vi "CheckforDFDToolkit.vi"(8 "error in (no error)":errorcluster) -> (0 "error out":errorcluster, 3 "NI LabVIEW Digital Filter Design Toolkit version":string)   [LabVIEW 2013]
uses:
  <vilib>/nisyscfg/Get Installed Components.vi
  <vilib>/nisyscfg/nisyscfg.lvlib
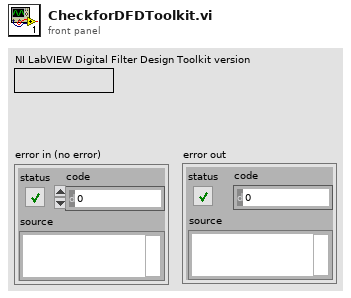
[diagram p1: front panel]
types:
  T1 = typedef "nisyscfg.lvlib/Software 1.2.ctl" = cluster{"title":string, "description":string, "ID":string, "version":string, "component type":T2}
  T2 = typedef "nisyscfg.lvlib/Component Type.ctl" = u32
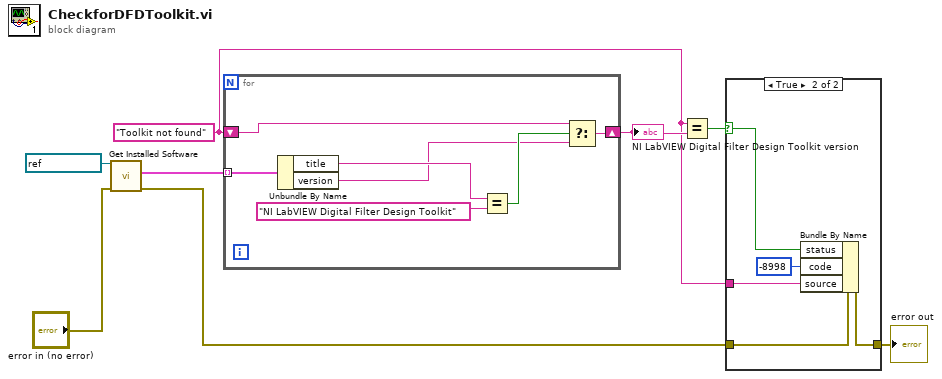
[diagram p0: block diagram]
diagram:
  w1 = "Toolkit not found" ("version")
  n1 = call-poly <vilib>:"Get Installed Software.vi"("error in (no error)"="error in (no error)", "Session in"=refnum<k21> "localhost") -> ("error out"=w3:errorcluster, "Software Components"=w7:T1[])  [unwired: 7 in, 1 out]
  n2 = for {
    tunnel: w7 -> [w15] mode=indexing
    shift-right: [w12] -> w6
    shift-left: w1 -> [w9]
    n3 = Unbundle By Name(w15) -> ("title"=w13:string, "version"=w10:string)
    n4 = Equal?(x=w13, y="NI LabVIEW Digital Filter Design Toolkit" ("regular expression")) -> (x = y?=w11:bool)
    n5 = Select(t=w9, s=w11, f=w10) -> (s? t:f=w12:string)
  }
  "NI LabVIEW Digital Filter Design Toolkit version" <- w6
  n6 = Equal?(x=w1, y=w6) -> (x = y?=w4:bool)
  n7 = case shown="True" w4 {
    selector: w4 -> [_ w19]
    tunnel: w3 -> [w16 w21]
    tunnel: [w16 w20] -> w2
    tunnel: w1 -> [_ w18]
    frame False {
    }
    frame True {
      n8 = Bundle By Name(cluster=w21, "status"=w19, "code"=-8998, "source"=w18) -> (w20:errorcluster)
    }
  }
  "error out" <- w2
